vi "Global_BOC (SubVI).vi"() -> ()   [LabVIEW 2017]
uses:
  Unicorn Labview Library/Control/paramUnicorn.ctl
  Unicorn Labview Library/Control/connectionParam.ctl
  Unicorn Labview Library/Control/JSONParam.ctl
panel:
  in  "Tab Control":enum32{"Connect", "Page 2"}(tab)
  in  "paramUnicorn":T1={"conParam"={"ReadIntParam"=TRUE, "ReadDescrParam"=FALSE, "ReadFloatParam"=TRUE, "debug"=FALSE, "ReadJSON"=TRUE, "IP_address"="192.168.1.216", "N_attempts"=3, "type_con"=enum."TCP", "MB_address"=1, "VISA"="COM1", "connection ID"=refnum, "nameDevices"="", "timeout"=3000, "port"=2000, "type_version"="0F0C0001", "baud_rate"=115200, "VersionControl"=TRUE, "TCP_conn"=TRUE}, "Param"={"ParamInt"=[["Режим работы", "", "", "", "", "", "ModeWork"], ["Режим сканирования", "", "Включение режима выполнения циклов сканирования", "", "", "", "CCEnable"], ["Количество тактов", "", "Количество тактов выполняемых в каждом цикле при включении режима сканирования", "32", "1", "%d", "CCTicksCount"], ["ФНЧ приемников", "МГц", "Частота среза фильтра низких частот приемников сигналов элементов ФЛ", "", "", "", "LPFilter"], ["ФВЧ приемников", "МГц", "Частота среза фильтра низких частот приемников сигналов элементов ФЛ", "", "", "", "HPFilter"], ["Тестирование цифрового интерфейса АЦП", "", "Передача по цифровому интерфейсу АЦП предустановленных или заданной пользователем последовательности данных", "", "", "", "PatternMode"], ["Тестовые данные 1 для АЦП", "", "Слово 1 данных задаваемое пользователем для тестирования цифрового интерфейса АЦП в режиме паттерна", "16383", "0", "%d", "PatternValue1"], ["Тестовые данные 2 для АЦП", "", "Слово 2 данных задаваемое пользователем для тестирования цифрового интерфейса АЦП в режиме паттерна", "16383", "0", "%d", "PatternValue2"], ["Номер такта для тестового захвата", "", "Номер такта для выполнения тестирования настроек выбранного такта ", "32", "1", "%d", "TestTickNum"], ["Амплитуда импульсов возбуждения ГИ №1 для каналов 1…8", "В", "Амплитуда импульсов возбуждения для ПЭП с 1 по 8", "", "", "", "Pulser1Level"], ["Амплитуда импульсов возбуждения ГИ №2 для каналов 9…16", "В", "Амплитуда импульсов возбуждения для ПЭП с 9 по 16", "", "", "", "Pulser2Level"], ["IP адрес электронного блока по умолчанию", "IPv4", "Присваивается электронному блоку если не был получен автоматически от DCHP сервера", "", "", "", "IPDefaultAddress"], ["Маска подсети", "IPv4", "Присваивается электронному блоку если не был получен автоматически от DCHP сервера", "", "", "", "IPDefaultNetMask"], ["Основной шлюз ", "IPv4", "Присваивается электронному блоку если не был получен автоматически от DCHP сервера", "", "", "", "IPDefaultGW"], ["Текущий IP адрес электронного блока", "IPv4", "Присваивается электронному блоку DCHP сервером", "", "", "", "IPCurrentAddress"], ["IP адрес для передачи UDP пакетов", "IPv4", "IP адрес на который будут отправляется информационные UDP пакеты", "", "", "", "IPAddressUDP"], ["Порт для передачи UDP пакетов от ГИ №1, каналы 1…8", "", "Порт, на который будут отправляется информационные UDP пакеты от ГИ №1, каналы 1…8", "65535", "0", "%d", "Port1UDP"], ["Порт для передачи UDP пакетов от ГИ №2, каналы 9…16", "", "Порт, на который будут отправляется информационные UDP пакеты от ГИ №2, каналы 9…16", "65535", "0", "%d", "Port2UDP"], ["Тип и версия ПЛИС №1", "", "Тип и версия встроенного ПО ПЛИС платы приема", "", "", "0x%08x", "IPFPGA1TypeVer"], ["Дата сборки ПО ПЛИС №1", "Date Time", "Дата сборки встроенного ПО ПЛИС платы приема", "", "", "%d", "IPFPGA1BuildTime"], ["Тип и версия ПЛИС №2", "", "Тип и версия встроенного ПО ПЛИС платы приема", "", "", "0x%08x", "IPFPGA2TypeVer"], ["Дата сборки ПО ПЛИС №2", "UNIX Time", "Дата сборки встроенного ПО ПЛИС платы приема", "", "", "%d", "IPFPGA2BuildTime"], ["Дата сборки ПО МК мониторинга", "UNIX Time", "Дата сборки ПО МК мониторинга платы приема", "", "", "%d", "IPADCMonMCUBuildTime"], ["Дата сборки ПО МК мониторинга ИП D2", "UNIX Time", "Дата сборки ПО МК мониторинга платы источника питания D2", "", "", "%d", "IPPMD2MCUBuildTime"], ["Дата сборки ПО МК мониторинга ИП D6", "UNIX Time", "Дата сборки ПО МК мониторинга платы источника питания D6", "", "", "%d", "IPPMD4MCUBuildTime"], ["Сохранение параметров", "", "Сохранение параметров в энергонезависимую память", "", "", "", "IPSaveParem"]], "ParamTelemetry"=[["Core uptime", "s", "", "", "", "%.1f", "CoreUptime"], ["FPGA №1 uptime", "s", "", "", "", "%.1f", "EP2C8time1"], ["FPGA №2 uptime", "s", "", "", "", "%.1f", "EP2C8time2"], ["TelStatusHF_EU", "", "", "0.01", "-0.01", "%.0f", "TelStatusHF_EU"], ["Энкодер №1", "мкм", "Текущее значение счетчика энкодера №1 модуля синхронизации", "", "", "%.0f", "TelEncoder1CurrData"], ["Счетчик импыльсов", "мкм", "Текущее значение счетчика импульсов модуля синхронизации", "", "", "%.0f", "TelPulseCurrData"], ["EncoderParam1", "мкм", "Значение поля «EncoderParam1» пакетов потока передачи данных", "", "", "%.0f", "TelEncoderParam1"], ["EncoderParam2", "мкм", "Значение поля «EncoderParam2» пакетов потока передачи данных", "", "", "%.0f", "TelEncoderParam2"], ["Tel33VDMON_G_min", "В", "", "", "", "%.3f", "Tel33VDMON_G_min"], ["Tel33VDMON_G_avg", "В", "", "", "", "%.3f", "Tel33VDMON_G_avg"], ["Tel33VDMON_G_max", "В", "", "", "", "%.3f", "Tel33VDMON_G_max"], ["_TelVMON_RB0_min", "В", "", "", "", "%.3f", "_TelVMON_RB0_min"], ["_TelVMON_RB0_avg", "В", "", "", "", "%.3f", "_TelVMON_RB0_avg"], ["_TelVMON_RB0_max", "В", "", "", "", "%.3f", "_TelVMON_RB0_max"], ["_TelVMON_PAB0_min", "В", "", "", "", "%.3f", "_TelVMON_PAB0_min"], ["_TelVMON_PAB0_avg", "В", "", "", "", "%.3f", "_TelVMON_PAB0_avg"], ["_TelVMON_PAB0_max", "В", "", "", "", "%.3f", "_TelVMON_PAB0_max"], ["_TelVMON_RB1_min", "В", "", "", "", "%.3f", "_TelVMON_RB1_min"], ["_TelVMON_RB1_avg", "В", "", "", "", "%.3f", "_TelVMON_RB1_avg"], ["_TelVMON_RB1_max", "В", "", "", "", "%.3f", "_TelVMON_RB1_max"], ["_TelVMON_PAB1_min", "В", "", "", "", "%.3f", "_TelVMON_PAB1_min"], ["_TelVMON_PAB1_avg", "В", "", "", "", "%.3f", "_TelVMON_PAB1_avg"], ["_TelVMON_PAB1_max", "В", "", "", "", "%.3f", "_TelVMON_PAB1_max"], ["PM D2 Uptime", "s", "", "", "", "%.0f", "TelPMD2Up_time"], ["TelPMD2CInMin", "A", "", "3.15", "0.1", "%.3f", "TelPMD2CInMin"], ["TelPMD2CInAVG", "A", "", "3.15", "0.1", "%.3f", "TelPMD2CInAVG"], ["TelPMD2CInMax", "A", "", "3.15", "0.1", "%.3f", "TelPMD2CInMax"], ["TelPMD2VInMin", "V", "", "14.0", "10.5", "%.3f", "TelPMD2VInMin"], ["TelPMD2VInAVG", "V", "", "14.0", "10.5", "%.3f", "TelPMD2VInAVG"], ["TelPMD2VInMax", "V", "", "14.0", "10.5", "%.3f", "TelPMD2VInMax"], ["TelPMD2PInMin", "W", "", "30.0", "1.0", "%.3f", "TelPMD2PInMin"], ["TelPMD2PInAVG", "W", "", "30.0", "1.0", "%.3f", "TelPMD2PInAVG"], ["TelPMD2PInMax", "W", "", "30.0", "1.0", "%.3f", "TelPMD2PInMax"], ["TelPMD2VRefIntMin", "V", "", "1.22", "1.18", "%.3f", "TelPMD2VRefIntMin"], ["TelPMD2VRefIntAVG", "V", "", "1.22", "1.18", "%.3f", "TelPMD2VRefIntAVG"], ["TelPMD2VRefIntMax", "V", "", "1.22", "1.18", "%.3f", "TelPMD2VRefIntMax"], ["TelPMD2ConvFreq", "Hz", "", "135.0e3", "120.0e3", "%.0f", "TelPMD2ConvFreq"], ["TelPMD2TempSensor", "°C", "", "80.0", "10.0", "%.1f", "TelPMD2TempSensor"], ["PM D6 Uptime", "s", "", "", "", "%.0f", "TelPMD6Up_time"], ["TelPMD6Vp27VMin", "V", "", "240.0", "200.0", "%.3f", "TelPMD6Vp27VMin"], ["TelPMD6Vp27VAVG", "V", "", "240.0", "200.0", "%.3f", "TelPMD6Vp27VAVG"], ["TelPMD6Vp27VMax", "V", "", "240.0", "200.0", "%.3f", "TelPMD6Vp27VMax"], ["TelPMD6Vp8VMin", "V", "", "9.5", "7.0", "%.3f", "TelPMD6Vp8VMin"], ["TelPMD6Vp8VAVG", "V", "", "9.5", "7.0", "%.3f", "TelPMD6Vp8VAVG"], ["TelPMD6Vp8VMax", "V", "", "9.5", "7.0", "%.3f", "TelPMD6Vp8VMax"], ["TelPMD6Vp5VMin", "V", "", "5.3", "4.8", "%.3f", "TelPMD6Vp5VMin"], ["TelPMD6Vp5VAVG", "V", "", "5.3", "4.8", "%.3f", "TelPMD6Vp5VAVG"], ["TelPMD6Vp5VMax", "V", "", "5.3", "4.8", "%.3f", "TelPMD6Vp5VMax"], ["TelPMD6Vp20VMin", "V", "", "19.0", "17.0", "%.3f", "TelPMD6Vp20VMin"], ["TelPMD6Vp20VAVG", "V", "", "19.0", "17.0", "%.3f", "TelPMD6Vp20VAVG"], ["TelPMD6Vp20VMax", "V", "", "19.0", "17.0", "%.3f", "TelPMD6Vp20VMax"], ["TelPMD6Vn8VMin", "V", "", "-7.0", "-9.5", "%.3f", "TelPMD6Vn8VMin"], ["TelPMD6Vn8VAVG", "V", "", "-7.0", "-9.5", "%.3f", "TelPMD6Vn8VAVG"], ["TelPMD6Vn8VMax", "V", "", "-7.0", "-9.5", "%.3f", "TelPMD6Vn8VMax"], ["TelPMD6Vn20VMin", "V", "", "22.0", "18.0", "%.3f", "TelPMD6Vn20VMin"], ["TelPMD6Vn20VAVG", "V", "", "22.0", "18.0", "%.3f", "TelPMD6Vn20VAVG"], ["TelPMD6Vn20VMax", "V", "", "22.0", "18.0", "%.3f", "TelPMD6Vn20VMax"], ["TelPMD6VRefIntMin", "V", "", "1.22", "1.18", "%.3f", "TelPMD6VRefIntMin"], ["TelPMD6VRefIntAVG", "V", "", "1.22", "1.18", "%.3f", "TelPMD6VRefIntAVG"], ["TelPMD6VRefIntMax", "V", "", "1.22", "1.18", "%.3f", "TelPMD6VRefIntMax"], ["TelPMD6TempSensor", "°C", "", "80.0", "10.0", "%.1f", "TelPMD6TempSensor"], ["TelPMPassPacketCount", "", "", "", "", "%.0f", "TelPMPassPacketCount"], ["TelPMErrorPacketCount", "", "", "", "", "%.0f", "TelPMErrorPacketCount"], ["_rb0_p_v_protection_min", "В", "", "5.5", "4.5", "%.3f", "_rb0_p_v_protection_min"], ["_rb0_p_v_protection_avg", "В", "", "5.5", "4.5", "%.3f", "_rb0_p_v_protection_avg"], ["_rb0_p_v_protection_max", "В", "", "5.5", "4.5", "%.3f", "_rb0_p_v_protection_max"], ["_rb0_p_5va_min", "В", "", "5.5", "4.5", "%.3f", "_rb0_p_5va_min"], ["_rb0_p_5va_avg", "В", "", "5.5", "4.5", "%.3f", "_rb0_p_5va_avg"], ["_rb0_p_5va_max", "В", "", "5.5", "4.5", "%.3f", "_rb0_p_5va_max"], ["_rb0_p_33vd_min", "В", "", "3.6", "3.0", "%.3f", "_rb0_p_33vd_min"], ["_rb0_p_33vd_avg", "В", "", "3.6", "3.0", "%.3f", "_rb0_p_33vd_avg"], ["_rb0_p_33vd_max", "В", "", "3.6", "3.0", "%.3f", "_rb0_p_33vd_max"], ["_rb0_p_18va_min", "В", "", "1.6", "2.0", "%.3f", "_rb0_p_18va_min"], ["_rb0_p_18va_avg", "В", "", "1.6", "2.0", "%.3f", "_rb0_p_18va_avg"], ["_rb0_p_18va_max", "В", "", "1.6", "2.0", "%.3f", "_rb0_p_18va_max"], ["_rb0_p_12vd_min", "В", "", "1.3", "1.1", "%.3f", "_rb0_p_12vd_min"], ["_rb0_p_12vd_avg", "В", "", "1.3", "1.1", "%.3f", "_rb0_p_12vd_avg"], ["_rb0_p_12vd_max", "В", "", "1.39", "1.1", "%.3f", "_rb0_p_12vd_max"], ["_rb0_m_5va_min", "В", "", "-4.5", "-5.5", "%.3f", "_rb0_m_5va_min"], ["_rb0_m_5va_avg", "В", "", "-4.5", "-5.5", "%.3f", "_rb0_m_5va_avg"], ["_rb0_m_5va_max", "В", "", "-4.5", "-5.5", "%.3f", "_rb0_m_5va_max"], ["_rb0_m_v_protection_min", "В", "", "-4.5", "-5.5", "%.3f", "_rb0_m_v_protection_min"], ["_rb0_m_v_protection_avg", "В", "", "-4.5", "-5.5", "%.3f", "_rb0_m_v_protection_avg"], ["_rb0_m_v_protection_max", "В", "", "-4.5", "-5.5", "%.3f", "_rb0_m_v_protection_max"], ["_rb0_control_point_min", "В", "", "", "", "%.3f", "_rb0_control_point_min"], ["_rb0_control_point_avg", "В", "", "", "", "%.3f", "_rb0_control_point_avg"], ["_rb0_control_point_max", "В", "", "", "", "%.3f", "_rb0_control_point_max"], ["_rb1_p_v_protection_min", "В", "", "5.5", "4.5", "%.3f", "_rb1_p_v_protection_min"], ["_rb1_p_v_protection_avg", "В", "", "5.5", "4.5", "%.3f", "_rb1_p_v_protection_avg"], ["_rb1_p_v_protection_max", "В", "", "5.5", "4.5", "%.3f", "_rb1_p_v_protection_max"], ["_rb1_p_5va_min", "В", "", "5.5", "4.5", "%.3f", "_rb1_p_5va_min"], ["_rb1_p_5va_avg", "В", "", "5.5", "4.5", "%.3f", "_rb1_p_5va_avg"], ["_rb1_p_5va_max", "В", "", "5.5", "4.5", "%.3f", "_rb1_p_5va_max"], ["_rb1_p_33vd_min", "В", "", "3.6", "3.0", "%.3f", "_rb1_p_33vd_min"], ["_rb1_p_33vd_avg", "В", "", "3.6", "3.0", "%.3f", "_rb1_p_33vd_avg"], ["_rb1_p_33vd_max", "В", "", "3.6", "3.0", "%.3f", "_rb1_p_33vd_max"], ["_rb1_p_18va_min", "В", "", "2.0", "1.6", "%.3f", "_rb1_p_18va_min"], ["_rb1_p_18va_avg", "В", "", "2.0", "1.6", "%.3f", "_rb1_p_18va_avg"], ["_rb1_p_18va_max", "В", "", "2.0", "1.6", "%.3f", "_rb1_p_18va_max"], ["_rb1_p_12vd_min", "В", "", "1.3", "1.1", "%.3f", "_rb1_p_12vd_min"], ["_rb1_p_12vd_avg", "В", "", "1.3", "1.1", "%.3f", "_rb1_p_12vd_avg"], ["_rb1_p_12vd_max", "В", "", "1.35", "1.1", "%.3f", "_rb1_p_12vd_max"], ["_rb1_m_5va_min", "В", "", "-4.5", "-5.5", "%.3f", "_rb1_m_5va_min"], ["_rb1_m_5va_avg", "В", "", "-4.5", "-5.5", "%.3f", "_rb1_m_5va_avg"], ["_rb1_m_5va_max", "В", "", "-4.5", "-5.5", "%.3f", "_rb1_m_5va_max"], ["_rb1_m_v_protection_min", "В", "", "-4.5", "-5.5", "%.3f", "_rb1_m_v_protection_min"], ["_rb1_m_v_protection_avg", "В", "", "-4.5", "-5.5", "%.3f", "_rb1_m_v_protection_avg"], ["_rb1_m_v_protection_max", "В", "", "-4.5", "-5.5", "%.3f", "_rb1_m_v_protection_max"], ["_rb1_control_point_min", "В", "", "", "", "%.3f", "_rb1_control_point_min"], ["_rb1_control_point_avg", "В", "", "", "", "%.3f", "_rb1_control_point_avg"], ["_rb1_control_point_max", "В", "", "", "", "%.3f", "_rb1_control_point_max"], ["_pab0_m_12v_min", "В", "", "-11.0", "-13.0", "%.3f", "_pab0_m_12v_min"], ["_pab0_m_12v_avg", "В", "", "-11.0", "-13.0", "%.3f", "_pab0_m_12v_avg"], ["_pab0_m_12v_max", "В", "", "-11.0", "-13.0", "%.3f", "_pab0_m_12v_max"], ["_pab0_m_20v_min", "В", "", "-18.0", "-22.0", "%.3f", "_pab0_m_20v_min"], ["_pab0_m_20v_avg", "В", "", "-18.0", "-22.0", "%.3f", "_pab0_m_20v_avg"], ["_pab0_m_20v_max", "В", "", "-18.0", "-22.0", "%.3f", "_pab0_m_20v_max"], ["_pab0_p_15v_min", "В", "", "16.5", "13.5", "%.3f", "_pab0_p_15v_min"], ["_pab0_p_15v_avg", "В", "", "16.5", "13.5", "%.3f", "_pab0_p_15v_avg"], ["_pab0_p_15v_max", "В", "", "16.5", "13.5", "%.3f", "_pab0_p_15v_max"], ["_pab0_p_5v_min", "В", "", "5.5", "4.5", "%.3f", "_pab0_p_5v_min"], ["_pab0_p_5v_avg", "В", "", "5.5", "4.5", "%.3f", "_pab0_p_5v_avg"], ["_pab0_p_5v_max", "В", "", "5.5", "4.5", "%.3f", "_pab0_p_5v_max"], ["_pab0_p_8v_min", "В", "", "8.8", "7.2", "%.3f", "_pab0_p_8v_min"], ["_pab0_p_8v_avg", "В", "", "8.8", "7.2", "%.3f", "_pab0_p_8v_avg"], ["_pab0_p_8v_max", "В", "", "8.8", "7.2", "%.3f", "_pab0_p_8v_max"], ["_pab0_p_hv_min", "В", "", "250.0", "10.0", "%.3f", "_pab0_p_hv_min"], ["_pab0_p_hv_avg", "В", "", "250.0", "10.0", "%.3f", "_pab0_p_hv_avg"], ["_pab0_p_hv_max", "В", "", "250.0", "10.0", "%.3f", "_pab0_p_hv_max"], ["_pab0_p_20v_min", "В", "", "22.0", "18.0", "%.3f", "_pab0_p_20v_min"], ["_pab0_p_20v_avg", "В", "", "22.0", "18.0", "%.3f", "_pab0_p_20v_avg"], ["_pab0_p_20v_max", "В", "", "22.0", "18.0", "%.3f", "_pab0_p_20v_max"], ["_pab0_p_220v_min", "В", "", "240.0", "200.0", "%.3f", "_pab0_p_220v_min"], ["_pab0_p_220v_avg", "В", "", "240.0", "200.0", "%.3f", "_pab0_p_220v_avg"], ["_pab0_p_220v_max", "В", "", "240.0", "200.0", "%.3f", "_pab0_p_220v_max"], ["_pab1_m_12v_min", "В", "", "-11.0", "-13.0", "%.3f", "_pab1_m_12v_min"], ["_pab1_m_12v_avg", "В", "", "-11.0", "-13.0", "%.3f", "_pab1_m_12v_avg"], ["_pab1_m_12v_max", "В", "", "-11.0", "-13.0", "%.3f", "_pab1_m_12v_max"], ["_pab1_m_20v_min", "В", "", "-18.0", "-22.0", "%.3f", "_pab1_m_20v_min"], ["_pab1_m_20v_avg", "В", "", "-18.0", "-22.0", "%.3f", "_pab1_m_20v_avg"], ["_pab1_m_20v_max", "В", "", "-18.0", "-22.0", "%.3f", "_pab1_m_20v_max"], ["_pab1_p_15v_min", "В", "", "16.5", "13.5", "%.3f", "_pab1_p_15v_min"], ["_pab1_p_15v_avg", "В", "", "16.5", "13.5", "%.3f", "_pab1_p_15v_avg"], ["_pab1_p_15v_max", "В", "", "16.5", "13.5", "%.3f", "_pab1_p_15v_max"], ["_pab1_p_5v_min", "В", "", "5.5", "4.5", "%.3f", "_pab1_p_5v_min"], ["_pab1_p_5v_avg", "В", "", "5.5", "4.5", "%.3f", "_pab1_p_5v_avg"], ["_pab1_p_5v_max", "В", "", "5.5", "4.5", "%.3f", "_pab1_p_5v_max"], ["_pab1_p_8v_min", "В", "", "8.8", "7.2", "%.3f", "_pab1_p_8v_min"], ["_pab1_p_8v_avg", "В", "", "8.8", "7.2", "%.3f", "_pab1_p_8v_avg"], ["_pab1_p_8v_max", "В", "", "8.8", "7.2", "%.3f", "_pab1_p_8v_max"], ["_pab1_p_hv_min", "В", "", "250.0", "10.0", "%.3f", "_pab1_p_hv_min"], ["_pab1_p_hv_avg", "В", "", "250.0", "10.0", "%.3f", "_pab1_p_hv_avg"], ["_pab1_p_hv_max", "В", "", "250.0", "10.0", "%.3f", "_pab1_p_hv_max"], ["_pab1_p_20v_min", "В", "", "22.0", "18.0", "%.3f", "_pab1_p_20v_min"], ["_pab1_p_20v_avg", "В", "", "22.0", "18.0", "%.3f", "_pab1_p_20v_avg"], ["_pab1_p_20v_max", "В", "", "22.0", "18.0", "%.3f", "_pab1_p_20v_max"], ["_pab1_p_220v_min", "В", "", "240.0", "200.0", "%.3f", "_pab1_p_220v_min"], ["_pab1_p_220v_avg", "В", "", "240.0", "200.0", "%.3f", "_pab1_p_220v_avg"], ["_pab1_p_220v_max", "В", "", "240.0", "200.0", "%.3f", "_pab1_p_220v_max"]], "ParamFloat"=[], "TableCount"=[[32, 9], [32, 9], [2, 1]], "NeedParamPrepare"=[], "NumParam"={"NTelem"=201, "NInt"=16, "NFloat"=10}, "NTable"=2}}
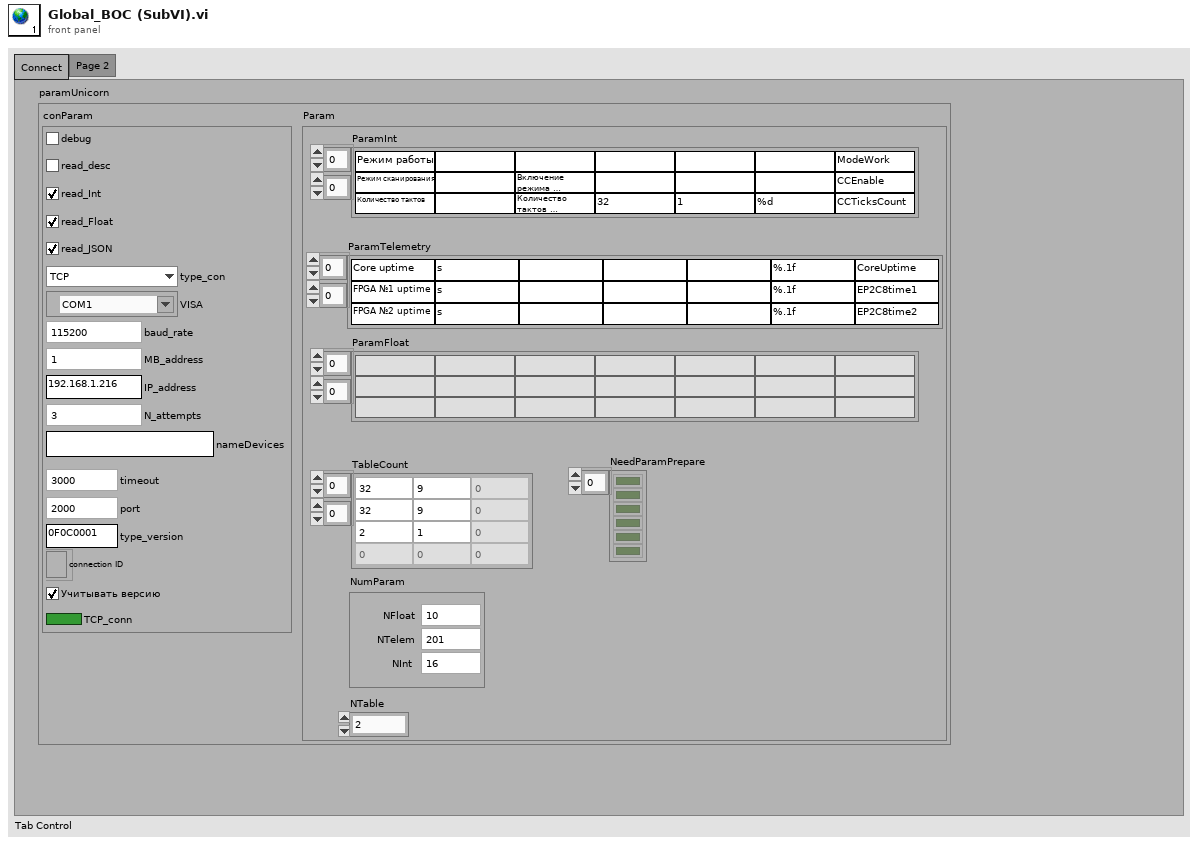
[diagram p1: front panel]
types:
  T1 = typedef "paramUnicorn.ctl" = cluster{"conParam":T2, "Param":T3}
  T2 = typedef "Unicorn Library.lvlib/connectionParam.ctl" = cluster{"ReadIntParam":bool, "ReadDescrParam":bool, "ReadFloatParam":bool, "debug":bool, "ReadJSON":bool, "IP_address":string, "N_attempts":i32, "type_con":enum16{"Serial", "TCP"}, "MB_address":i32, "VISA":refnum<visa-resource-name>, "connection ID":refnum<k5>, "nameDevices":string, "timeout":i32, "port":u16, "type_version":string, "baud_rate":u32, "VersionControl":bool, "TCP_conn":bool}
  T3 = typedef "Unicorn Library.lvlib/JSONParam.ctl" = cluster{"ParamInt":string[][], "ParamTelemetry":string[][], "ParamFloat":string[][], "TableCount":i32[][], "NeedParamPrepare":bool[], "NumParam":cluster{"NTelem":i32, "NInt":i32, "NFloat":i32}, "NTable":i32}
diagram:
